vi "ServerTCPIP_Autoguider2016.vi"() -> ()   [LabVIEW 2018]
panel:
  in  "stop":bool
  out "Status":string
  out "TCP/IP 2":bool
  out "connection ID 2":refnum<k5>
  out "serial ref":refnum<visa-resource-name>
  out "Command":string
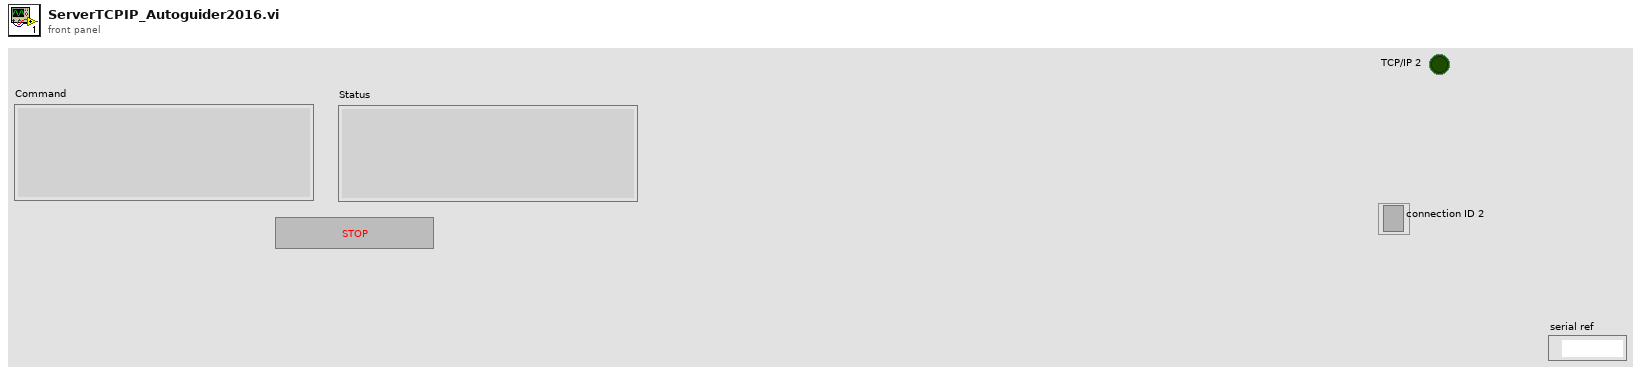
[diagram p1: front panel]
types:
  T1 = enum16{"Standard", "Buffered", "CRLF", "Immediate"}
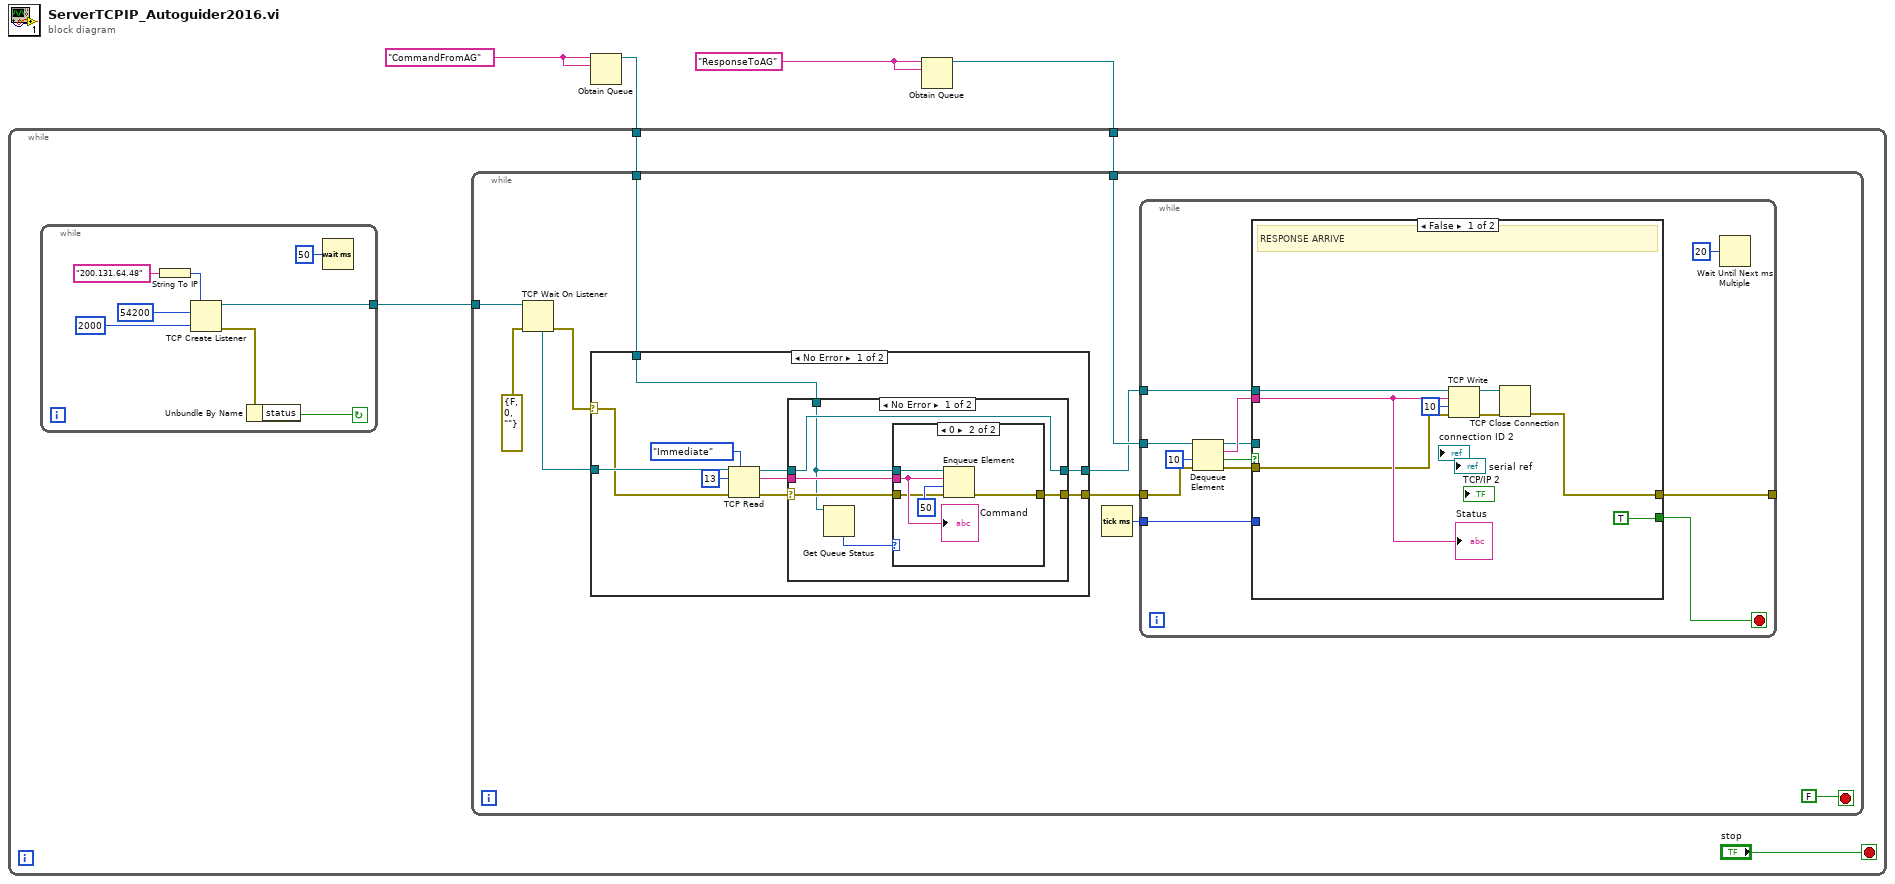
[diagram p0: block diagram]
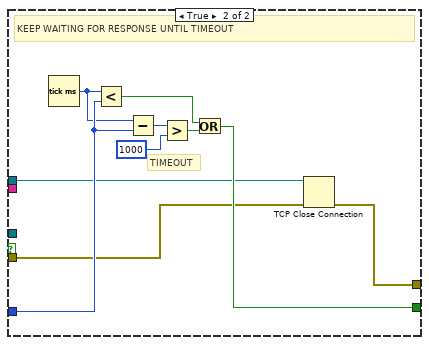
[diagram p2: hidden frame]
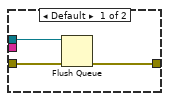
[diagram p3: hidden frame]
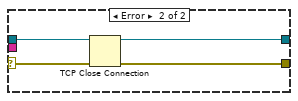
[diagram p4: hidden frame]
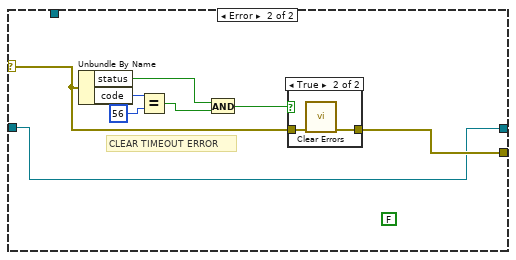
[diagram p5: hidden frame]
diagram:
  w2 = "ResponseToAG" ("name (unnamed)")
  w3 = "CommandFromAG" ("name (unnamed)")
  n1 = Obtain Queue(name (unnamed)=w3, element data type=w3) -> (queue out=w4:refnum<queue>)  [unwired: 3 in, 2 out]
  n2 = Obtain Queue(name (unnamed)=w2, element data type=w2) -> (queue out=w1:refnum<queue>)  [unwired: 3 in, 2 out]
  n3 = while {
    tunnel: w4 -> [w7]
    tunnel: w1 -> [w6]
    stop <- "stop" stop-if-true
    n4 = while {
      tunnel: [w89] -> w8
      stop <- w90 continue-if-true
      n5 = String To IP(1:"200.131.64.48" ("name")) -> (0:w94:u32)
      n6 = TCP Create Listener(7:w94, 9:2000 ("timeout ms (25000)"), 10:u16 54200 ("port")) -> (0:w91:errorcluster, 3:w89:refnum<k5>)  [unwired: 2 in, 1 out]
      n7 = Unbundle By Name(w91) -> ("status"=w90:bool)
      n8 = Wait (ms)(milliseconds to wait=u32 50) -> ()  [unwired: 1 out]
    }
    n9 = while {
      tunnel: w8 -> [w18]
      tunnel: w7 -> [w15]
      tunnel: w6 -> [w12]
      stop <- FALSE stop-if-true
      n10 = TCP Wait On Listener(8:errorcluster {"status"=FALSE, "code"=0, "source"=""} ("error in (no error)"), 11:w18) -> (0:w16:errorcluster, 4:w17:refnum<k5>)  [unwired: 2 in, 3 out]
      n11 = case shown="No Error" w16 {
        selector: w16 -> [w51 w79]
        tunnel: w17 -> [w54 w77]
        tunnel: [w52 w78] -> w13
        tunnel: w15 -> [w53 _]
        tunnel: [w50 w77] -> w11
        frame No Error {
          n12 = TCP Read(connection ID=w54, bytes to read=13, error in (no error)=w51, 7:T1."Immediate" ("mode (standard)")) -> (connection ID out=w57:refnum<k5>, data out=w56:string, error out=w55:errorcluster)  [unwired: 1 in]
          n13 = case shown="No Error" w55 {
            selector: w55 -> [w61 w76]
            tunnel: w53 -> [w60 _]
            tunnel: [w64 w74] -> w52
            tunnel: w57 -> [w62 w75]
            tunnel: w56 -> [w63 _]
            tunnel: [w62 w73] -> w50
            frame No Error {
              n14 = Get Queue Status(queue=w60) -> (# elements in queue=w59:i32)  [unwired: 2 in, 7 out]
              n15 = case shown="0" w59 {
                tunnel: [w65 w72] -> w64
                tunnel: w63 -> [_ w71]
                tunnel: w61 -> [w66 w69]
                tunnel: w60 -> [w67 w68]
                frame Default {
                  n16 = Flush Queue(queue=w67, error in (no error)=w66) -> (error out=w65:errorcluster)  [unwired: 2 out]
                }
                frame 0 {
                  n17 = Enqueue Element(queue=w68, element=w71, timeout in ms (-1)=50, error in (no error)=w69) -> (error out=w72:errorcluster)  [unwired: 2 out]
                  "Command" <- w71
                }
              }
            }
            frame Error {
              n18 = TCP Close Connection(connection ID=w75, error in (no error)=w76) -> (connection ID out=w73:refnum<k5>, error out=w74:errorcluster)  [unwired: 1 in]
            }
          }
        }
        frame Error {
          (unwired) FALSE
          # "CLEAR TIMEOUT ERROR"
          n19 = Unbundle By Name(w79) -> ("status"=w80:bool, "code"=w84:i32)
          n20 = Equal?(x=w84, y=56 ("specific error code to clear (0: all)")) -> (x = y?=w81:bool)
          n21 = And(x=w80, y=w81) -> (x .and. y?=w82:bool)
          n22 = case shown="True" w82 {
            tunnel: w79 -> [w85 w87]
            tunnel: [w85 w86] -> w78
            frame False {
            }
            frame True {
              n23 = call <vilib>:"Clear Errors.vi"("error in (no error)"=w87) -> ("error out"=w86:errorcluster)  [unwired: 5 in, 1 out]
            }
          }
        }
      }
      n24 = Tick Count (ms)() -> (millisecond timer value=w14:u32)
      n25 = while {
        tunnel: w14 -> [w26]
        tunnel: w12 -> [w23]
        tunnel: w11 -> [w22]
        tunnel: w13 -> [w25]
        tunnel: [w24] -> _
        stop <- w27 stop-if-true
        n26 = Dequeue Element(queue=w23, timeout in ms (-1)=10, error in (no error)=w25) -> (queue out=w19:refnum<queue>, element=w30:string, timed out?=w29:bool, error out=w28:errorcluster)
        n27 = case shown="False" w29 {
          tunnel: w28 -> [w31 w41]
          tunnel: w30 -> [w36 _]
          tunnel: w26 -> [_ w48]
          tunnel: [TRUE w42] -> w27
          tunnel: [w38 w40] -> w24
          tunnel: w22 -> [w33 w39]
          tunnel: w19 -> [_ _]
          frame False {
            # "RESPONSE ARRIVE"
            n28 = TCP Write(connection ID=w33, data in=w36, error in (no error)=w31, 9:10 ("timeout ms (25000)")) -> (connection ID out=w34:refnum<k5>, error out=w35:errorcluster)  [unwired: 1 out]
            n29 = TCP Close Connection(connection ID=w34, error in (no error)=w35) -> (error out=w38:errorcluster)  [unwired: 1 in, 1 out]
            "Status" <- w36
          }
          frame True {
            # "TIMEOUT"
            # "KEEP WAITING FOR RESPONSE UNTIL TIMEOUT"
            n30 = Tick Count (ms)() -> (millisecond timer value=w47:u32)
            n31 = Less?(x=w47, y=w48) -> (x < y?=w43:bool)
            n32 = Subtract(x=w47, y=w48) -> (x-y=w46:u32)
            n33 = Greater?(x=w46, y=u32 1000 ("millisecond timer value")) -> (0:w44:bool)
            n34 = Or(x=w43, y=w44) -> (x .or. y?=w42:bool)
            n35 = TCP Close Connection(connection ID=w39, error in (no error)=w41) -> (error out=w40:errorcluster)  [unwired: 1 in, 1 out]
          }
        }
        n36 = Wait Until Next ms Multiple(millisecond multiple=u32 20) -> ()  [unwired: 1 out]
      }
    }
  }
